vi "Event UI.vi"(8 "error in (no error)":errorcluster, 10 "ContextData In":refnum<class "ContextData.lvclass">, 11 "Wait Event in":refnum<class "Wait Event.lvclass">) -> (0 "error out":errorcluster, 3 "Wait Event out":refnum<class "Wait Event.lvclass">)   [LabVIEW 2019, in "Wait Event.lvclass"]
uses:
  Wait Event.lvclass
  ContextData/ContextData.lvclass
  Context/Context.lvclass
  User State 1/User State 1.lvclass
  C:/Users/Felipe-PC/Documents/Projetos/Projetos Github/OOP-State-Machine/State/State.lvclass
  ContextData/ContextData.lvclass/ContextData.ctl
  User State 2/User State 2.lvclass
  Exit/Exit.lvclass
panel:
  in  "Do Something Else <Replace Me>":bool
  in  "Do Something <Replace Me>":bool
  in  "Exit":bool
  # "These controls have associated \"Value Changed\" events configured in the Event Structure on the diagram.\n\nReplace them (and reconfigure the Event Structure) with the controls you need for your application."
  # "This template is for the Simple State Machine design pattern.\n\nSee the block diagram for more information on how to use this template."
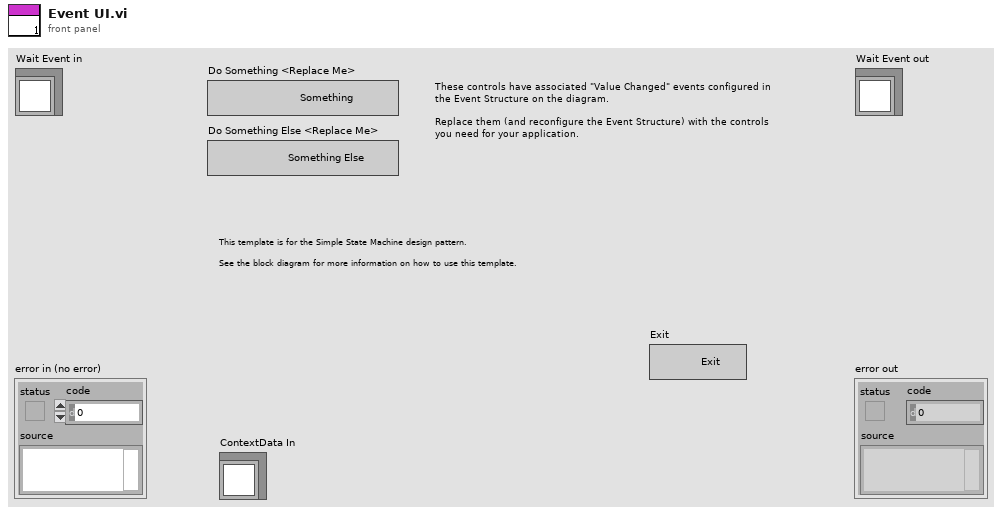
[diagram p1: front panel]
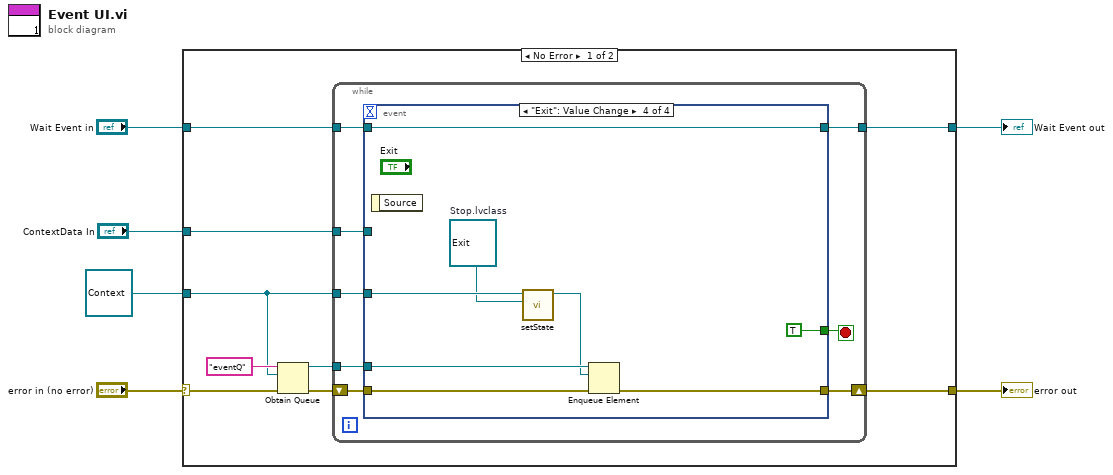
[diagram p0: block diagram]
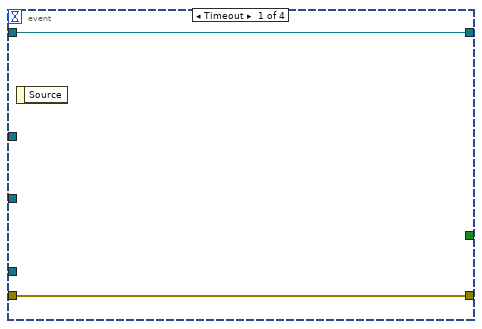
[diagram p2: hidden frame]
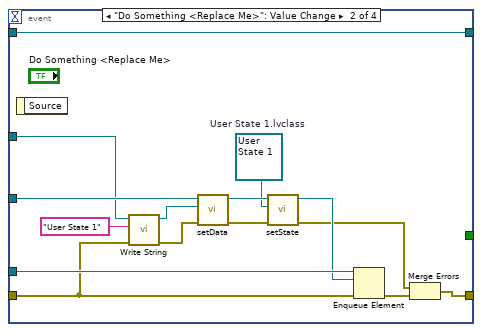
[diagram p3: hidden frame]
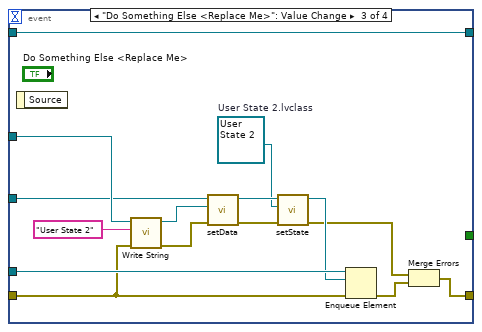
[diagram p4: hidden frame]
diagram:
  n1 = case shown="No Error" "error in (no error)" {
    selector: "error in (no error)" -> [w13 w65]
    tunnel: [w12 w65] -> w5
    tunnel: [w14 w64] -> w3
    tunnel: "Wait Event in" -> [w15 w64]
    tunnel: refnum<class "Context.lvclass"> refnum ("Context.lvclass") -> [w8 _]
    tunnel: "ContextData In" -> [w7 _]
    frame No Error {
      n2 = Obtain Queue(name (unnamed)="eventQ", element data type=w8, error in (no error)=w13) -> (queue out=w9:refnum<queue>, error out=w11:errorcluster)  [unwired: 2 in, 1 out]
      n3 = while {
        tunnel: w15 -> [w23]
        tunnel: [w22] -> w14
        shift-right: [w20] -> w12
        shift-left: w11 -> [w21]
        tunnel: w9 -> [w19]
        tunnel: w8 -> [w17]
        tunnel: w7 -> [w16]
        stop <- w18 stop-if-true
        n4 = event shown="[3] \"Exit\": Value Change" {
          selector: _ -> [_ _ _ _]
          dyn-events: _ -> [_ _ _ _]
          timeout: _ -> [_ _ _ _]
          tunnel: w23 -> [w25 w40 w55 w63]
          tunnel: [w25 w40 w55 w63] -> w22
          tunnel: w21 -> [w24 w27 w44 w62]
          tunnel: [w24 w28 w42 w61] -> w20
          tunnel: w19 -> [_ w38 w53 w60]
          tunnel: [_ _ _ TRUE] -> w18
          tunnel: w17 -> [_ w36 w47 w58]
          tunnel: w16 -> [_ w32 w48 _]
          event Timeout {
            n5 = event-data() -> ()  [unwired: 1 in, 1 out]
          }
          event "Do Something <Replace Me>": Value Change {
            w34 = refnum<class "User State 1.lvclass"> refnum  # User State 1.lvclass
            n6 = event-data() -> ()  [unwired: 1 in, 1 out]
            n7 = call "Write String.vi"("error in (no error)"=w27, "String <Replace Me>"="User State 1", "ContextData in"=w32) -> ("error out"=w33:errorcluster, "ContextData out"=w29:refnum<class "ContextData.lvclass">)  [unwired: 7 in]
            n8 = call "setData.vi"("error in (no error)"=w33, "ContextData.lvclass"=w29, "Context in"=w36) -> ("error out"=w37:errorcluster, "Context out"=w35:refnum<class "Context.lvclass">)  [unwired: 7 in]
            n9 = call "setState.vi"("error in (no error)"=w37, "State.lvclass"=w34, "Context in"=w35) -> ("error out"=w26:errorcluster, "Context out"=w30:refnum<class "Context.lvclass">)  [unwired: 7 in]
            n10 = Enqueue Element(queue=w38, element=w30, error in (no error)=w27) -> (error out=w39:errorcluster)  [unwired: 1 in, 2 out]
            n11 = Merge Errors(w26, w39) -> (w28:errorcluster)
          }
          event "Do Something Else <Replace Me>": Value Change {
            w46 = refnum<class "User State 2.lvclass"> refnum  # User State 2.lvclass
            n12 = event-data() -> ()  [unwired: 1 in, 1 out]
            n13 = call "Write String.vi"("error in (no error)"=w44, "String <Replace Me>"="User State 2", "ContextData in"=w48) -> ("error out"=w50:errorcluster, "ContextData out"=w43:refnum<class "ContextData.lvclass">)  [unwired: 7 in]
            n14 = call "setData.vi"("error in (no error)"=w50, "ContextData.lvclass"=w43, "Context in"=w47) -> ("error out"=w52:errorcluster, "Context out"=w51:refnum<class "Context.lvclass">)  [unwired: 7 in]
            n15 = call "setState.vi"("error in (no error)"=w52, "State.lvclass"=w46, "Context in"=w51) -> ("error out"=w41:errorcluster, "Context out"=w45:refnum<class "Context.lvclass">)  [unwired: 7 in]
            n16 = Enqueue Element(queue=w53, element=w45, error in (no error)=w44) -> (error out=w54:errorcluster)  [unwired: 1 in, 2 out]
            n17 = Merge Errors(w41, w54) -> (w42:errorcluster)
          }
          event "Exit": Value Change {
            w57 = refnum<class "Exit.lvclass"> refnum  # Stop.lvclass
            n18 = event-data() -> ()  [unwired: 1 in, 1 out]
            n19 = call "setState.vi"("State.lvclass"=w57, "Context in"=w58) -> ("Context out"=w56:refnum<class "Context.lvclass">)  [unwired: 8 in, 1 out]
            n20 = Enqueue Element(queue=w60, element=w56, error in (no error)=w62) -> (error out=w61:errorcluster)  [unwired: 1 in, 2 out]
          }
        }
      }
    }
    frame Error {
    }
  }
  "error out" <- w5
  "Wait Event out" <- w3
